vi "Convert Complex Cluster to Magnitude.vi"(0 "IQ data (complex) In":cluster{"t0":dbl, "dt":dbl, "Y":cdb[]}={"t0"=0.0, "dt"=1.0, "Y"=[]} {"Y" format="%.2f"; "dt" format="%.2f"; "t0" format="%.2f"}, 7 "Public.Units":enum8{"Vrms", "dBm"}(ring), 11 "Error In":errorcluster) -> (4 "Magnitude Out":cluster{"t0":dbl, "dt":dbl, "Y":dbl[]}={"t0"=0.0, "dt"=1.0, "Y"=[]} {"Y" min=0.0 max=127.0 format="%.6f"; "dt" format="%.2f"; "t0" format="%.2f"}, 15 "Error Out":errorcluster)   [LabVIEW 2019]
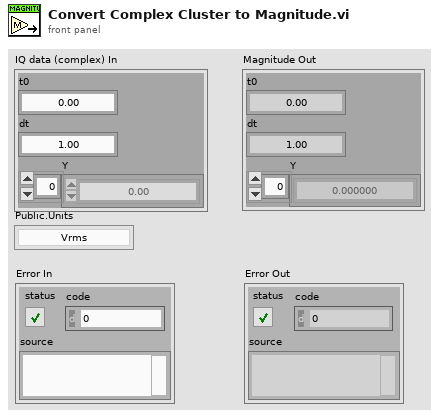
[diagram p1: front panel]
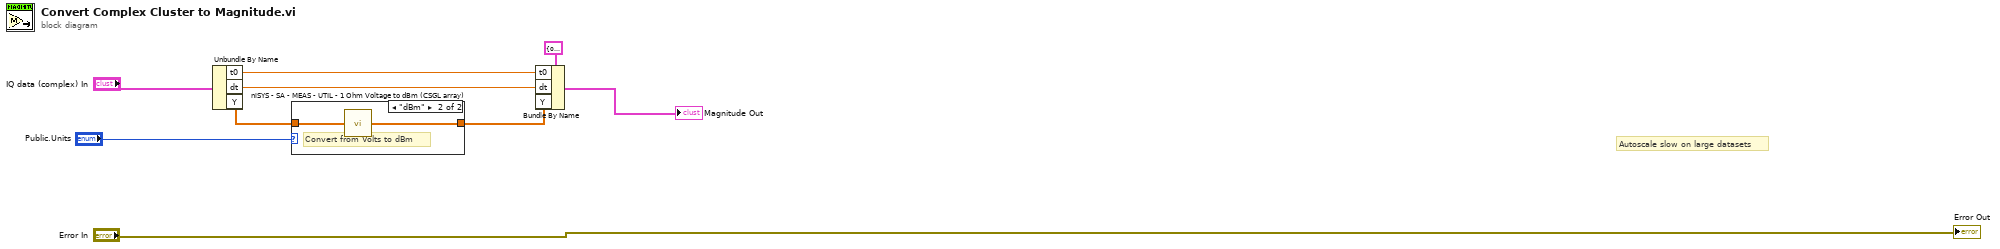
[diagram p0: block diagram]
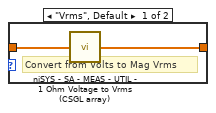
[diagram p2: hidden frame]
diagram:
  # "Autoscale slow on large datasets"
  n1 = Unbundle By Name("IQ data (complex) In") -> ("t0"=w6:dbl, "dt"=w5:dbl, "Y"=w2:cdb[])
  n2 = case shown="\"dBm\"" "Public.Units" {
    tunnel: w2 -> [w11 w13]
    tunnel: [w10 w12] -> w3
    frame "Vrms", Default {
      # "Convert from Volts to Mag Vrms"
      n3 = call "niSYS - SA - MEAS - UTIL - 1 Ohm Voltage to Vrms (CSGL array).vi"("Complex Array, V"=w11) -> ("Real Array, dBm"=w10:dbl[])  [unwired: 14 in]
    }
    frame "dBm" {
      # "Convert from Volts to dBm"
      n4 = call "niSYS - SA - MEAS - UTIL - 1 Ohm Voltage to dBm (CSGL array).vi"("Complex Array, V"=w13) -> ("Real Array, dBm"=w12:dbl[])  [unwired: 14 in]
    }
  }
  n5 = Bundle By Name(cluster=cluster{"t0":dbl, "dt":dbl, "Y":dbl[]} {"t0"=0.0, "dt"=1.0, "Y"=[]} ("Magnitude Out"), "t0"=w6, "dt"=w5, "Y"=w3) -> (→"Magnitude Out":cluster{"t0":dbl, "dt":dbl, "Y":dbl[]})
  "Error Out" <- "Error In"
